vi "Slow Down Tolerance.vi"(0 "Current Height":dbl, 1 "Lower Slow Down Tolerance":dbl, 5 "Upper Slow Down Tolerance":dbl, 7 "Max Height":dbl, 9 "Elevator Power":dbl, 11 "Slow Down Multiplier":dbl, 12 "Climb":bool) -> (6 "Motor Out":dbl)   [LabVIEW 2017]
panel:
  # "DISABLED"
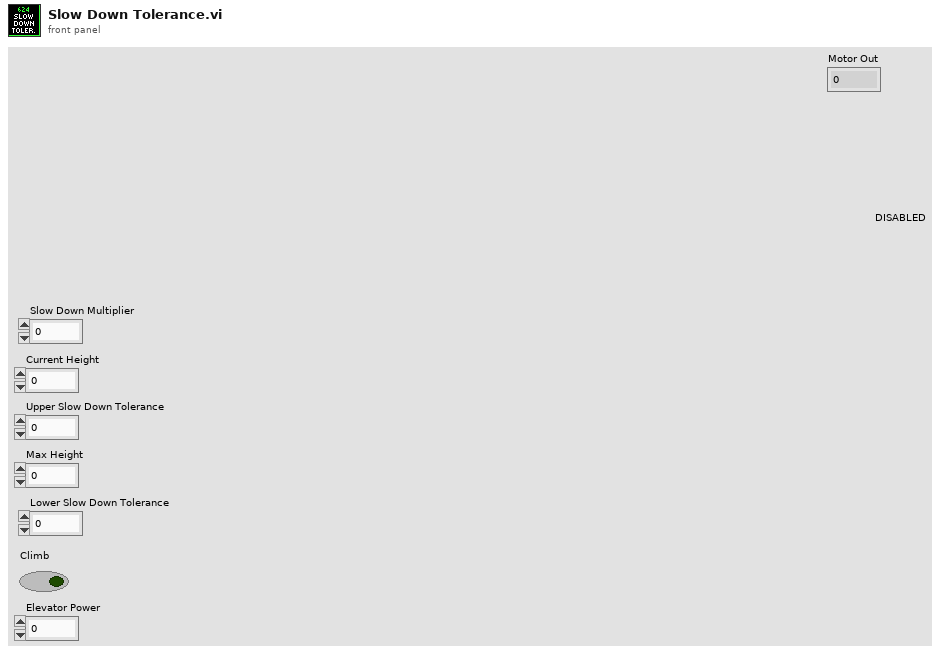
[diagram p1: front panel]
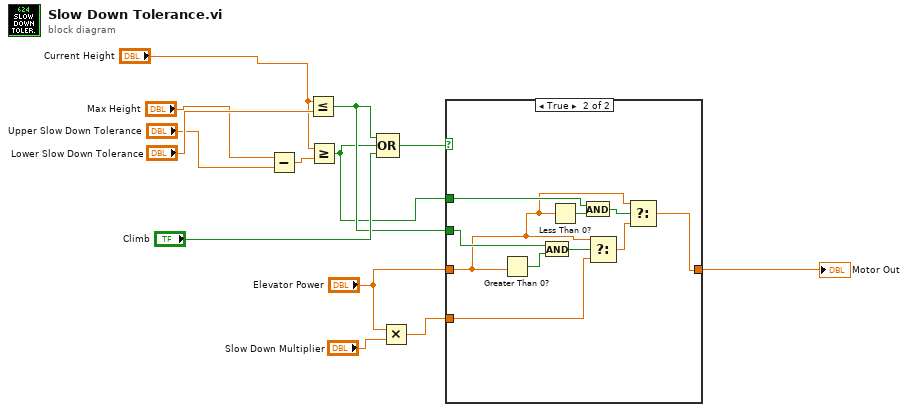
[diagram p0: block diagram]
diagram:
  n1 = Subtract(x="Max Height", y="Upper Slow Down Tolerance") -> (x-y=w12:dbl)
  n2 = Less Or Equal?(x="Current Height", y="Lower Slow Down Tolerance") -> (x <= y?=w2:bool)
  n3 = Greater Or Equal?(x="Current Height", y=w12) -> (x >= y?=w1:bool)
  n4 = Compound Arithmetic op=OR(w2, w1, "Climb") -> (w6:bool)
  n5 = Multiply(x="Elevator Power", y="Slow Down Multiplier") -> (x*y=w3:dbl)
  n6 = case shown="True" w6 {
    tunnel: "Elevator Power" -> [w14 w16]
    tunnel: [w14 w15] -> w8
    tunnel: w3 -> [_ w21]
    tunnel: w2 -> [_ w23]
    tunnel: w1 -> [_ w19]
    frame False {
    }
    frame True {
      n7 = Greater Than 0?(x=w16) -> (x > 0?=w24:bool)
      n8 = And(x=w23, y=w24) -> (x .and. y?=w22:bool)
      n9 = Less Than 0?(x=w16) -> (x < 0?=w20:bool)
      n10 = And(x=w19, y=w20) -> (x .and. y?=w18:bool)
      n11 = Select(t=w16, s=w22, f=w21) -> (s? t:f=w17:dbl)
      n12 = Select(t=w16, s=w18, f=w17) -> (s? t:f=w15:dbl)
    }
  }
  "Motor Out" <- w8
